vi "mhk_motor_data_int-diff.vi"() -> ()   [LabVIEW 2010]
uses:
  <vilib>/Analysis/2dsp.llb/Integral Method.ctl
  <vilib>/Utility/file.llb/Read From Spreadsheet File (DBL).vi
  <vilib>/Analysis/8numeric.llb/1D Numeric Integration.vi
  <vilib>/Analysis/NI_AALPro.lvlib
panel:
  out "size(s)":i32[](array[numeric])=[3, 15000]
  out "all rows":dbl[][](array[numeric]) format="%0.5f"
  out "delta x":dbl=0.0005
  in  "derivative method":u16(ring) items=["2nd Order Central", "4th Order Central", "Forward", "Backward"]
  out "dX/dt":dbl[](array[numeric])
  out "response vector":dbl[](array[numeric])
  out "Integral X":dbl[](array[numeric])
  out "response\nvector\nsize":i32=15000
  out "1D integration\nresult":dbl=13.059835 format="%0.5f"
  out "Running Integral Graph":cluster{"Lower limit \"a\"":dbl, dbl, dbl[][]}(graph)={"Lower limit \"a\""=0.0, 0.0005, array2x15000[30000 elements]}
  in  "Plot BG Color":bool
  out "Approx. Integral \nover entire range\ndone en masse":dbl=13.05983499999999
  out "Function Graph":cluster{"Lower limit \"a\"":dbl, dbl, dbl[][]}(graph)={"Lower limit \"a\""=0.0, 0.0005, array2x15000[30000 elements]}
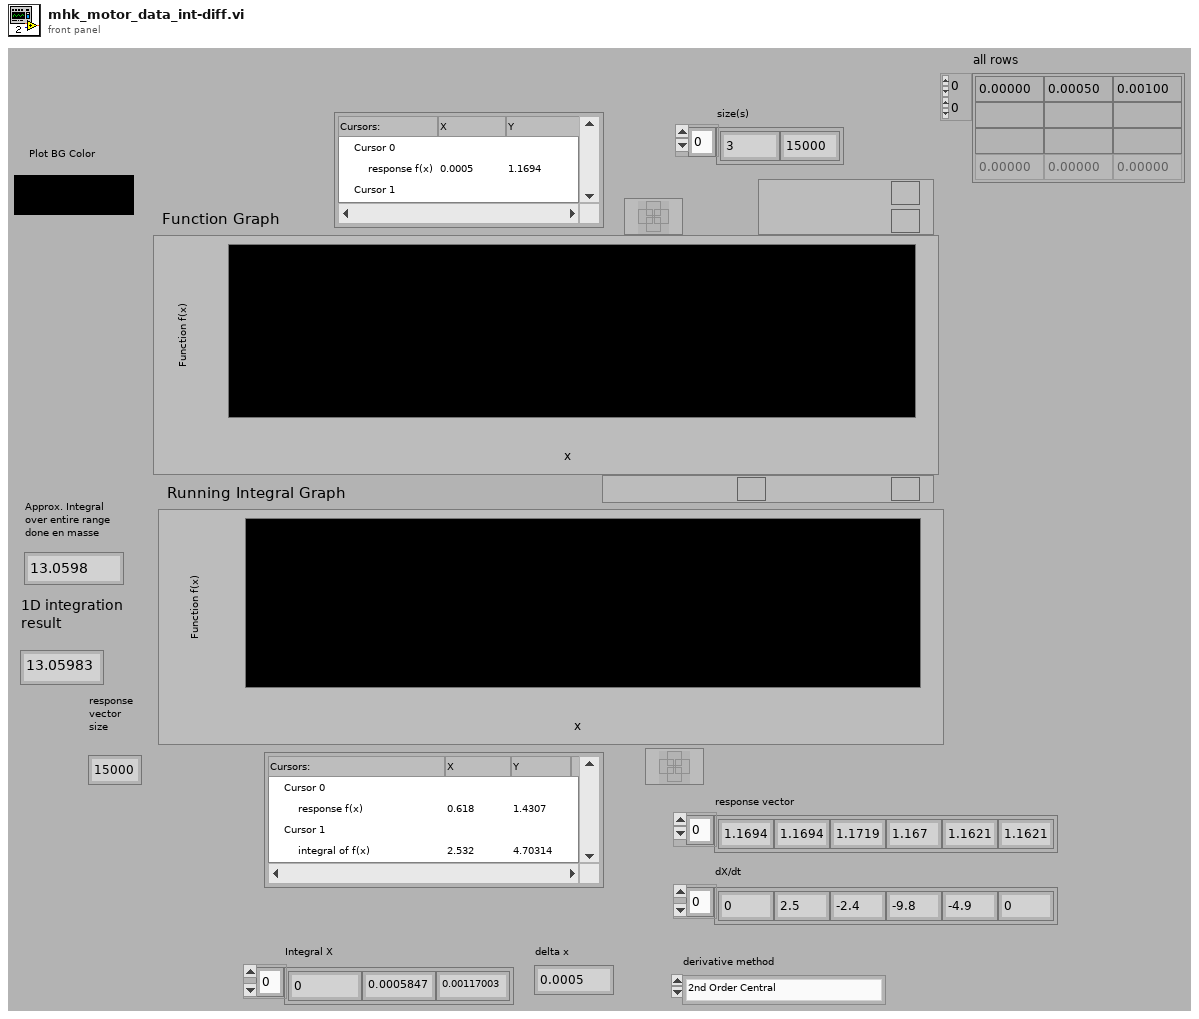
[diagram p1: front panel]
types:
  T1 = typedef "NI_AALPro.lvlib/Integral Method.ctl" = i32
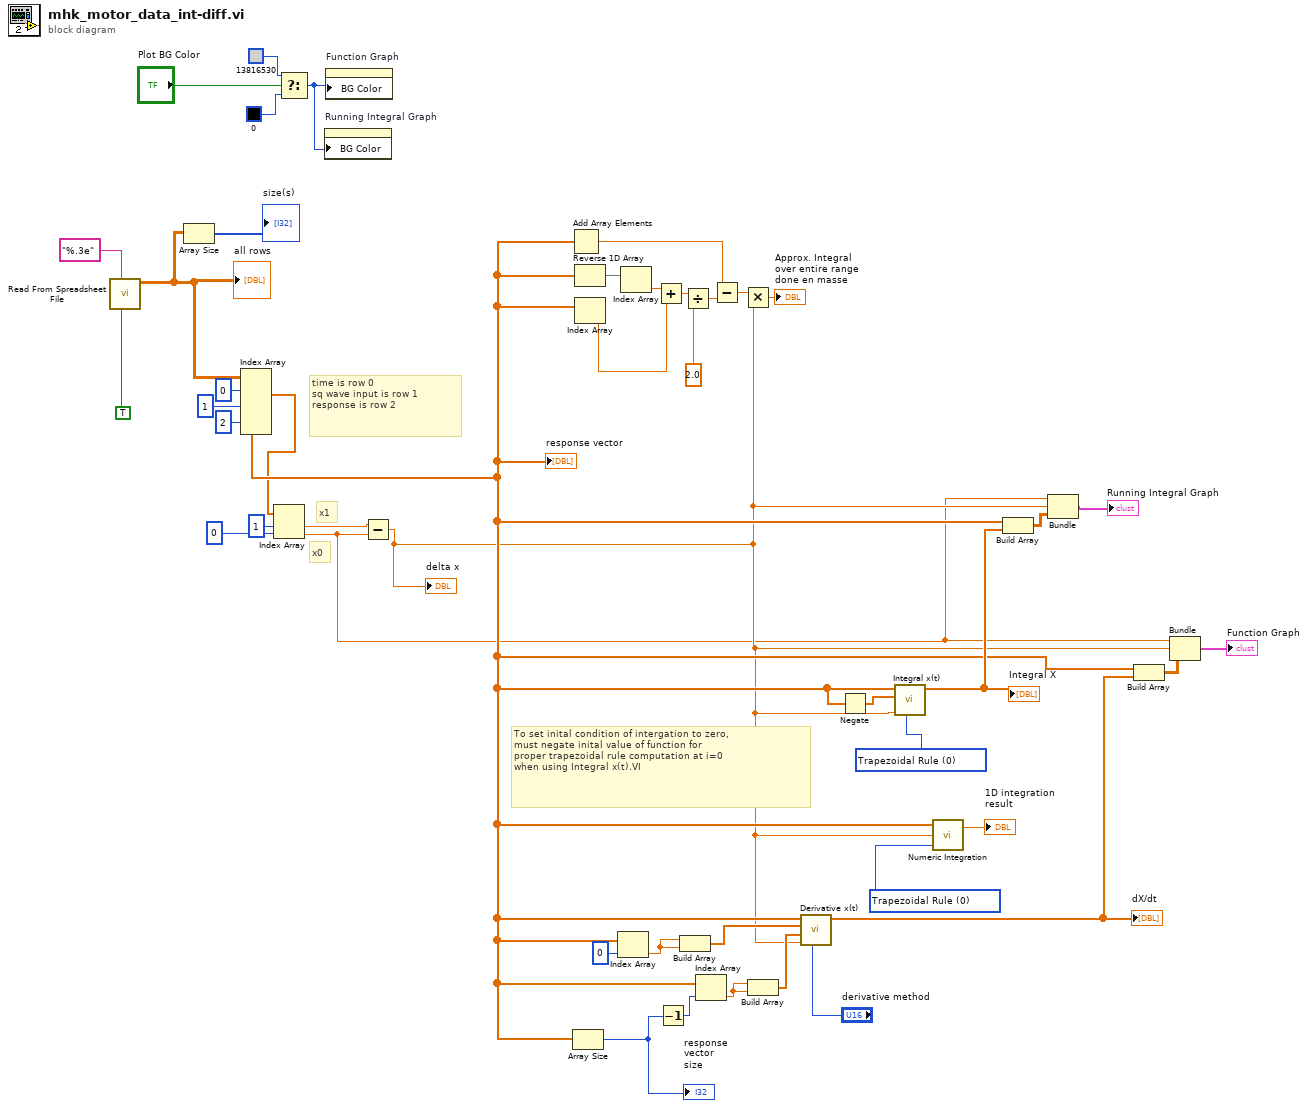
[diagram p0: block diagram]
diagram:
  w27 = T1 0 items=["Trapezoidal Rule", "Simpson's Rule", "Simpson's 3/8 Rule", "Bode Rule"] ("integration method")
  w29 = T1 0 items=["Trapezoidal Rule", "Simpson's Rule", "Simpson's 3/8 Rule", "Bode Rule"] ("integration method")
  # "time is row 0\nsq wave input is row 1\nresponse is row 2"
  # "x1"
  # "x0"
  # "To set inital condition of intergation to zero,\nmust negate inital value of function for \nproper trapezoidal rule computation at i=0 \nwhen using Integral x(t).VI"
  n1 = call-poly <vilib>:"Read From Spreadsheet File.vi"("transpose (no:F)"=TRUE, "format (%.3f)"="%.3e") -> ("all rows"=w12:dbl[][])  [unwired: 5 in, 4 out]
  "all rows" <- w12
  n2 = Array Size(array=w12) -> (size(s)=→"size(s)":i32[])
  n3 = Index Array(array=w12, index (row) #1=0 ("index (row)"), index (row) #2=1 ("index (row)"), index (row) #3=2 ("index (row)")) -> (element #1=w6:dbl[], element #3=w8:dbl[])  [unwired: 3 in, 1 out]
  "response vector" <- w8
  n4 = Index Array(array=w6, index #1=1 ("index"), index #2=0 ("index")) -> (element #1=w3:dbl, element #2=w1:dbl)
  n5 = Select(t=u32 13816530, s="Plot BG Color", f=u32 0) -> (s? t:f=w31:u32)
  n6 = property on="Running Integral Graph" class="WFGraph (strict)"("BG Color"=w31) -> ()  [unwired: 2 in, 2 out]
  n7 = property on="Function Graph" class="WFGraph (strict)"("BG Color"=w31) -> ()  [unwired: 2 in, 2 out]
  n8 = Subtract(x=w3, y=w1) -> (x-y=w2:dbl)
  "delta x" <- w2
  n9 = Add Array Elements(numeric array=w8) -> (sum=w38:dbl)
  n10 = Array Size(array=w8) -> (size(s)=w20:i32)
  "response\nvector\nsize" <- w20
  n11 = Reverse 1D Array(array=w8) -> (reversed array=w44:dbl[])
  n12 = Index Array(array=w8) -> (element=w42:dbl)  [unwired: 1 in]
  n13 = Index Array(array=w8, index=0) -> (element=w22:dbl)
  n14 = Index Array(array=w44) -> (element=w43:dbl)  [unwired: 1 in]
  n15 = Add(x=w43, y=w42) -> (x+y=w41:dbl)
  n16 = Decrement(x=w20) -> (x-1=w19:i32)
  n17 = Build Array(w22, w22) -> (w21:dbl[])
  n18 = Divide(x=w41, y=2.0) -> (x/y=w39:dbl)
  n19 = Index Array(array=w8, index=w19) -> (element=w18:dbl)
  n20 = Subtract(x=w38, y=w39) -> (x-y=w37:dbl)
  n21 = Multiply(x=w37, y=w2) -> (x*y=→"Approx. Integral \nover entire range\ndone en masse":dbl)
  n22 = Build Array(w18, w18) -> (w17:dbl[])
  n23 = call <vilib>:"Derivative x(t).vi"("method"="derivative method", "dt"=w2, "Final Condition"=w17, "Initial Condition"=w21, "X"=w8) -> ("dX/dt"=w16:dbl[])  [unwired: 5 in, 1 out]
  "dX/dt" <- w16
  n24 = Negate(x=w8) -> (-x=w24:dbl[])
  n25 = call <vilib>:"Integral x(t).vi"("integration method"=w27, "dt"=w2, "Initial Condition"=w24, "X"=w8) -> ("Integral X"=w25:dbl[])  [unwired: 6 in, 1 out]
  "Integral X" <- w25
  n26 = call-poly <vilib>:"Numeric Integration.vi"("integration method"=w29, "dt"=w2, "Input Array"=w8) -> ("result"=→"1D integration\nresult":dbl)  [unwired: 1 out]
  n27 = Build Array(w8, w25) -> (w30:dbl[][])
  n28 = Bundle(w1, w2, w30) -> (→"Running Integral Graph":cluster{dbl, dbl, dbl[][]})  [unwired: 1 in]
  n29 = Build Array(w8, w16) -> (w15:dbl[][])
  n30 = Bundle(w1, w2, w15) -> (→"Function Graph":cluster{dbl, dbl, dbl[][]})  [unwired: 1 in]
